vi "Module Type.vi"(11 "ValveControlModule in":refnum<class "DigitalControlModule.lvclass">) -> (2 "Module Type":string)   [LabVIEW 2020, in "VolatusControl.lvlib" / "DigitalControlModule.lvclass"]
uses:
  DigitalControlModule.lvclass
  DigitalControlModule.lvclass/DigitalControlModule.ctl
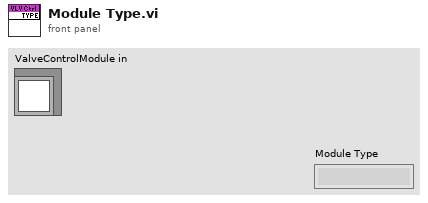
[diagram p1: front panel]
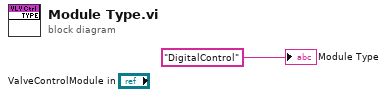
[diagram p0: block diagram]
diagram:
  "Module Type" <- "DigitalControl" ("Module Type")
